vi "Insert Subpanel UI.vi"(8 "error in (no error)":errorcluster, 10 "Subpanel in":refnum<vi>, 11 "LabVIEW Object":refnum<class>) -> (0 "error out":errorcluster, 2 "Subpanel out":refnum<vi>, 3 "LabVIEW Object out":refnum<class>)   [LabVIEW 2012]
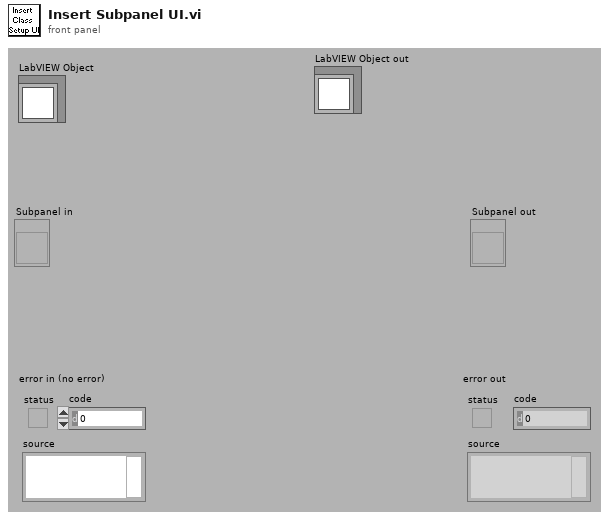
[diagram p1: front panel]
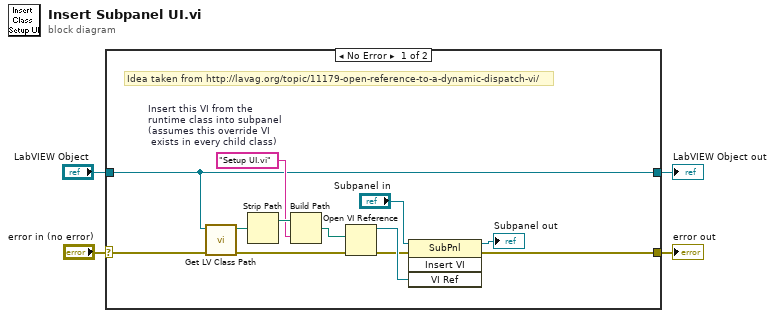
[diagram p0: block diagram]
diagram:
  n1 = case shown="No Error" "error in (no error)" {
    selector: "error in (no error)" -> [w16 w18]
    tunnel: [w15 w18] -> w3
    tunnel: "LabVIEW Object" -> [w5 w17]
    tunnel: [w5 w17] -> w1
    frame No Error {
      w12 = "Setup UI.vi"  # Insert this VI from the runtime class into subpanel (assumes this override VI   exists in every child class)
      # "Idea taken from http://lavag.org/topic/11179-open-reference-to-a-dynamic-dispatch-vi/"
      n2 = call <vilib>:"Get LV Class Path.vi"("error in (no error)"=w16, "object"=w5) -> ("error out"=w6:errorcluster, "class path"=w14:path)  [unwired: 8 out]
      n3 = Strip Path(path=w14) -> (stripped path=w13:path)  [unwired: 1 out]
      n4 = Build Path(base path=w13, name or relative path=w12) -> (appended path=w11:path)
      n5 = Open VI Reference(vi path=w11, error in (no error)=w6) -> (vi reference=w8:refnum<vi>, error out=w7:errorcluster)  [unwired: 4 out]
      n6 = invoke on="Invoke Node" class="SubPnl" method="Insert VI"(reference="Subpanel in", error in=w7, "VI Ref"=w8) -> (reference out=→"Subpanel out":refnum<vi>, error out=w15:errorcluster)  [unwired: 1 in, 2 out]
    }
    frame Error {
    }
  }
  "error out" <- w3
  "LabVIEW Object out" <- w1
